vi "MultiChannel LockIn Engine.vi"(7 "Lock-in Configuration":T1={"Type"=enum."FIR", "TC (s)"=1.0, "Filter \nRolloff"=enum."20 dB", "Order"=1} {"Order" min=1 step=1; "TC (s)" format="%.3p"}, 8 "Apply Change":bool, 9 "Sampling Rate":dbl, 10 "Signals":dbl[][](array[numeric]), 11 "Reference Signal":dbl[](array[numeric])) -> (0 "Theta":dbl[](array[numeric])=[0.08733391919393045] format="%.5f", 1 "R":dbl[](array[numeric])=[9.700001176496645] format="%.5f", 2 "X":dbl[](array[numeric])=[9.663032692990507] format="%.5f", 3 "Y":dbl[](array[numeric])=[0.8460626443904347] format="%.5f", 4 "Lock error":i32, 5 "Frequency":dbl=102.40333431899356 format="%.2f")   [LabVIEW 2020]
uses:
  Lockin Configuration.ctl
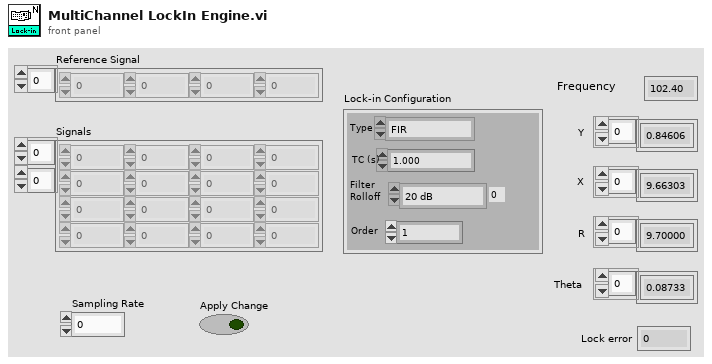
[diagram p1: front panel]
types:
  T1 = typedef "Lockin Configuration.ctl" = cluster{"Type":enum16{"IIR (2-dig)", "IIR (5-dig)", "FIR", "FIR (ENBW)", "FIR (Sync)"}, "TC (s)":dbl, "Filter \nRolloff":enum16{"20 dB", "40 dB", "60 dB", "80 dB", "100 dB", "120 dB", "140 dB", "160 dB", "180 dB", "200 dB"}, "Order":u32}
  T2 = enum16{"IIR (2-dig)", "IIR (5-dig)", "FIR", "FIR (ENBW)", "FIR (Sync)"}
  T3 = enum16{"20 dB", "40 dB", "60 dB", "80 dB", "100 dB", "120 dB", "140 dB", "160 dB", "180 dB", "200 dB"}
  T4 = enum16{"Reserved", "Sine", "Square", "Sine (sync)"}
  T5 = cluster{"fr":dbl, "Phase":dbl, "Order":u32, "Updated":bool, "Block Size":i32, "fs":dbl}
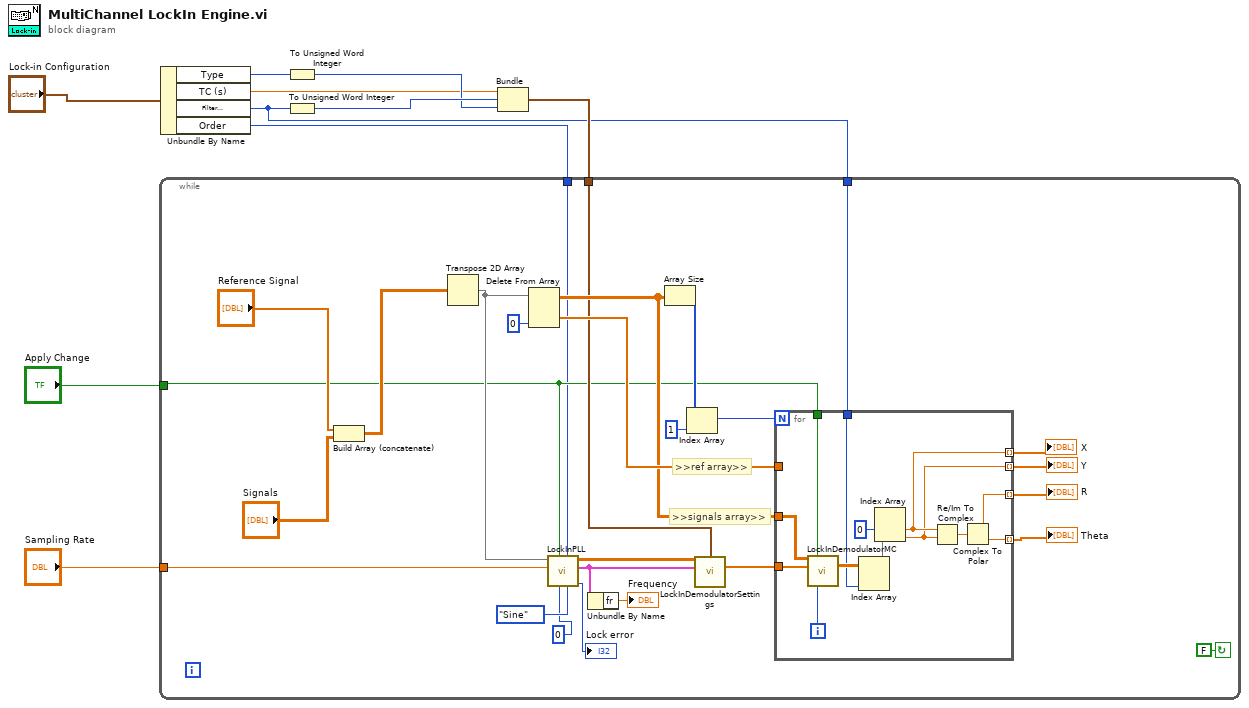
[diagram p0: block diagram]
diagram:
  n1 = Unbundle By Name("Lock-in Configuration") -> ("Type"=w5:T2, "TC (s)"=w4:dbl, "Filter \nRolloff"=w3:T3, "Order"=w2:u32)
  n2 = To Unsigned Word Integer(number=w5) -> (unsigned 16bit integer=w9:u16)
  n3 = To Unsigned Word Integer(number=w3) -> (unsigned 16bit integer=w10:u16)
  n4 = Bundle("TC (s)"=w4, w10, w9) -> (w8:cluster{"TC (s)":dbl, u16, u16})  [unwired: 1 in]
  n5 = while {
    tunnel: w3 -> [w34]
    tunnel: w8 -> [w20]
    tunnel: "Apply Change" -> [w13]
    tunnel: "Sampling Rate" -> [w12]
    tunnel: w2 -> [w11]
    stop <- FALSE ("stop") continue-if-true
    # ">>ref array>>"
    # ">>signals array>>"
    n6 = Build Array (concatenate)("Reference Signal", "Signals") -> (w16:dbl[][])
    n7 = Transpose 2D Array(2D array=w16) -> (transposed array=w19:dbl[][])
    n8 = Delete From Array(array=w19, index (col)=0 ("disabled index (col)")) -> (deleted portion=w26:dbl[], array with subset deleted=w25:dbl[][])  [unwired: 2 in]
    n9 = call "LockInPLL.vi"("Function"=T4."Sine", "Order"=w11, "Data Column"=u32 0, "Init"=w13, "fs"=w12, "Signal (in)"=w19) -> ("Lock error"=→"Lock error":i32, "Reference Info"=w22:T5, "Signal (out)"=w23:sgl[][])  [unwired: 2 in, 1 out]
    n10 = Unbundle By Name(w22) -> ("fr"=→"Frequency":dbl)
    n11 = Array Size(array=w25) -> (size(s)=w37:i32[])
    n12 = Index Array(array=w37, index=1) -> (element=w35:i32)
    n13 = call "LockInDemodulatorSettings.vi"("Signal (in)"=w23, "LP Filter Info"=w20, "Reference Info"=w22) -> ("LP Filter Settings"=w21:dbl[])  [unwired: 9 in, 3 out]
    n14 = for {
      N: w35 -> [_]
      tunnel: w13 -> [w50]
      tunnel: w34 -> [w46]
      tunnel: w26 -> [_]
      tunnel: w25 -> [w39]
      tunnel: [w44] -> w33 mode=indexing
      tunnel: [w43] -> w32 mode=indexing
      tunnel: [w42] -> w31 mode=indexing
      tunnel: [w41] -> w30 mode=indexing
      tunnel: w21 -> [w40]
      i -> [w38]
      n15 = call "LockInDemodulatorMC.vi"("Signal (in)"=w39, "Apply"=w50, "LP Filter Settings"=w40, "Data Column"=w38) -> ("Data (out)"=w47:dbl[][])  [unwired: 9 in, 2 out]
      n16 = Index Array(array=w47, index (col)=w46) -> (element=w49:dbl[])  [unwired: 1 in]
      n17 = Index Array(array=w49, index #1=0 ("index")) -> (element #1=w44:dbl, element #2=w43:dbl)  [unwired: 1 in]
      n18 = Re/Im To Complex(1:w43, 2:w44) -> (0:w45:cdb)
      n19 = Complex To Polar(r * e^(i*theta)=w45) -> (r=w42:dbl, theta=w41:dbl)
    }
    "X" <- w33
    "Y" <- w32
    "R" <- w31
    "Theta" <- w30
  }
